vi "PAM Sample Rate.vi"() -> ()   [LabVIEW 2020, in "PAM Library.lvlib"]
uses:
  PAM Library.lvlib
panel:
  in  "PAM Sample Rate":i32=64000
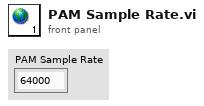
[diagram p1: front panel]
diagram:
